vi "NavigatorInputPrimitive.vi"(0 "error in":errorcluster, 2 "Component":T2, 3 "node":string) -> (1 "error out":errorcluster, 4 "Navigator Inputs":T1)   [LabVIEW 2012]
doc: "This VI gets the status of the Navigator Buttons"
uses:
  <userlib>/ROSforLV/ROS/Code/SubVIs/BaxterButtons.ctl
  <userlib>/ROSforLV/ROS/Code/Console/Servers/ServerSubs/TopicDef.ctl
  <userlib>/ROSforLV/ROS/Code/SubVIs/_ROSDirection.ctl
panel:
  out "Reply":string
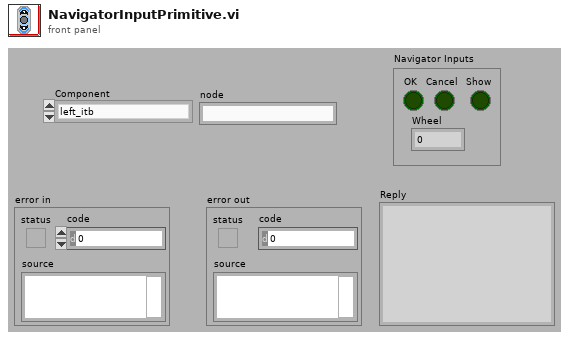
[diagram p1: front panel]
types:
  T1 = cluster{"OK":bool, "Cancel":bool, "Show":bool, "Wheel":u8}
  T2 = typedef "BaxterButtons.ctl" = enum16{"left_itb", "right_itb", "torso_left_itb", "torso_right_itb"}
  T3 = typedef "TopicDef.ctl" = cluster{"Topic":string, "Type":string, "Action":T4, "Update (ms)":u16, "write queue":u16}
  T4 = typedef "_ROSDirection.ctl" = enum16{"Node", "Publisher", "Subscriber", "Service Client"}
  T5 = typedef "_ROSControl.ctl" = cluster{"topic port":u16, "Node":string, "topic":string, "type":string, "node port":u16, "error ":errorcluster, "Direction":T4, "APIs":string[], "Update (ms)":u16, "write queue":u16}
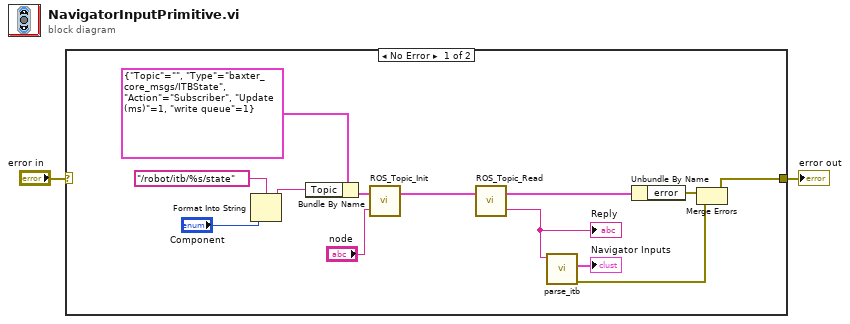
[diagram p0: block diagram]
diagram:
  n1 = case shown="No Error" "error in" {
    selector: "error in" -> [_ w16]
    tunnel: [w3 w16] -> w2
    frame No Error {
      n2 = Format Into String(format string="/robot/itb/%s/state" ("topic"), "Component") -> (resulting string=w10:string)  [unwired: 2 in, 1 out]
      n3 = Bundle By Name(cluster=T3 {"Topic"="", "Type"="baxter_core_msgs/ITBState", "Action"=enum."Subscriber", "Update (ms)"=1, "write queue"=1} ("Definitions"), "Topic"=w10) -> (w6:T3)
      n4 = call <userlib>:"ROS_Topic_Init.vi"("node"="node", "Definitions"=w6) -> ("ROS out"=w14:T5)  [unwired: 1 in]
      n5 = call <userlib>:"ROS_Topic_Read.vi"("ROS in"=w14) -> ("Reply"=w12:string, "ROS out"=w13:T5)  [unwired: 1 in]
      "Reply" <- w12
      n6 = call <userlib>:"parse_itb.vi"("msg in"=w12) -> ("error out"=w4:errorcluster, "Navigator Inputs"=→"Navigator Inputs":T1)  [unwired: 4 in, 1 out]
      n7 = Unbundle By Name(w13) -> ("error"=w5:errorcluster)
      n8 = Merge Errors(w5, w4) -> (w3:errorcluster)
    }
    frame Error {
    }
  }
  "error out" <- w2
